vi "Top Flywheel PID.vi"(10 "Top RPM":dbl, 11 "setpoint":dbl format="%.2f") -> (3 "output":dbl format="%.2f")   [LabVIEW 2016]
uses:
  <vilib>/addons/control/pid/pid.llb/PID (DBL).vi
  <vilib>/addons/control/pid/NI_PID_pid.lvlib
panel:
  out "Output":dbl(graph)
  out "RPM":dbl(graph)
  in  "PID gains":T1={"proportional gain (Kc)"=1e-08, "integral time (Ti, min)"=5e-07, "derivative time (Td, min)"=0.0} {"derivative time (Td, min)" format="%.9f"; "integral time (Ti, min)" format="%.10f"; "proportional gain (Kc)" format="%.10f"}
  in  "reinitialize? (F)":bool
  in  "output range":cluster{"output high":dbl, "output low":dbl}={"output high"=1.0, "output low"=0.0} {"output low" format="%.2f"; "output high" format="%.2f"}
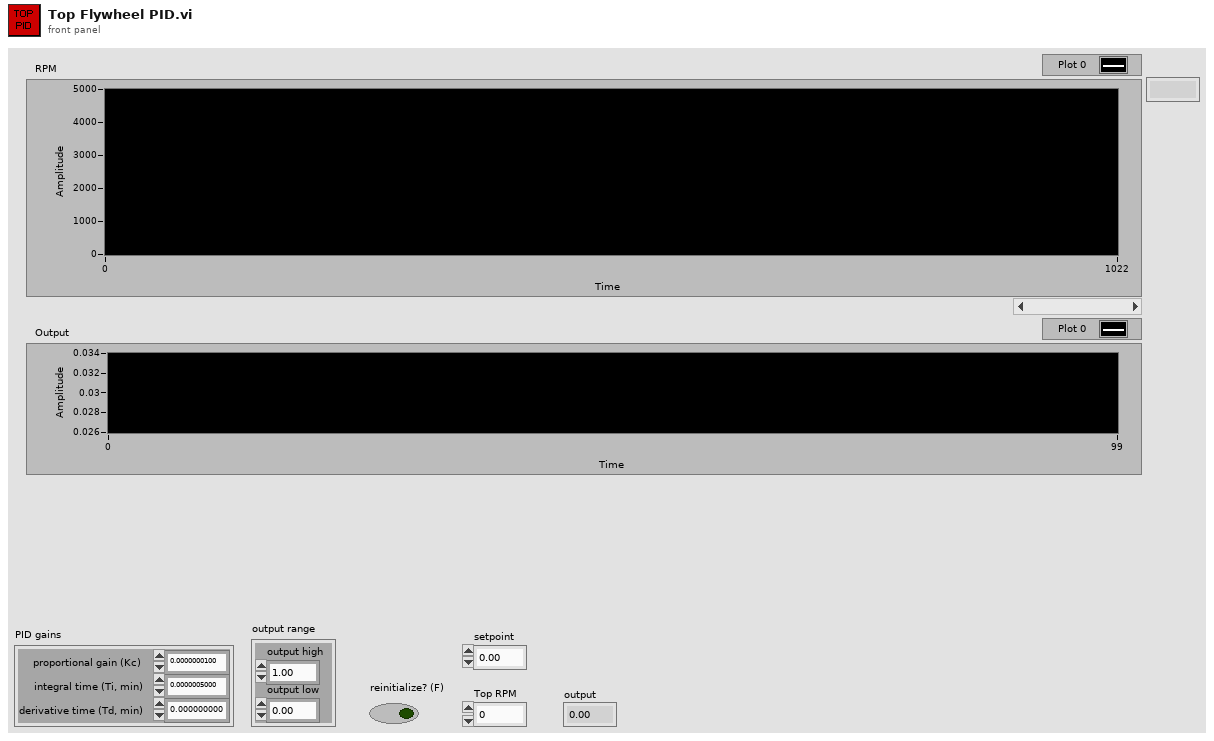
[diagram p1: front panel]
types:
  T1 = cluster{"proportional gain (Kc)":dbl, "integral time (Ti, min)":dbl, "derivative time (Td, min)":dbl}
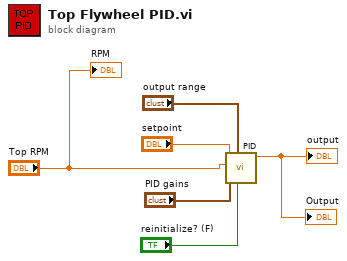
[diagram p0: block diagram]
diagram:
  n1 = call-poly <vilib>:"PID.vi"("reinitialize? (F)"="reinitialize? (F)", "output range"="output range", "PID gains"="PID gains", "process variable"="Top RPM", "setpoint"="setpoint") -> ("output"=→"output" →"Output":dbl)  [unwired: 5 in, 1 out]
  "RPM" <- "Top RPM"
